vi "3_datatypes.vi"() -> ()   [LabVIEW 2024]
uses:
  class/CalibReport/CalibReport.lvclass
  <vilib>/Python/Open Venv Python Session.vi
panel:
  in  "Datatypes":T1(tab)
  in  "input string":string
  out "result":string
  out "Boolean Output":bool
  in  "Input":bool
  out "Error from python":errorcluster
  in  "List Input":i32[](array[numeric])=[1, 2, 3, 4, 5]
  out "return list":i32[](array[numeric])
  in  "Map":map{string, i32}(c390)
  out "<JSON>":string
  out "CalibPoints":cluster{dbl[], dbl[]}(graph)
  out "__str__ from python object":string
  in  "Temperature [°C]":dbl
  in  "Stop":bool
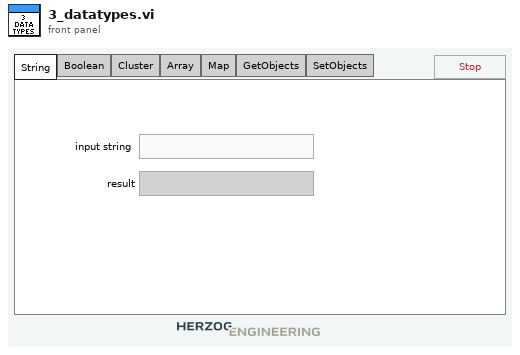
[diagram p1: front panel]
types:
  T1 = enum32{"String", "Boolean", "Cluster", "Array", "Map", "GetObjects", "SetObjects"}
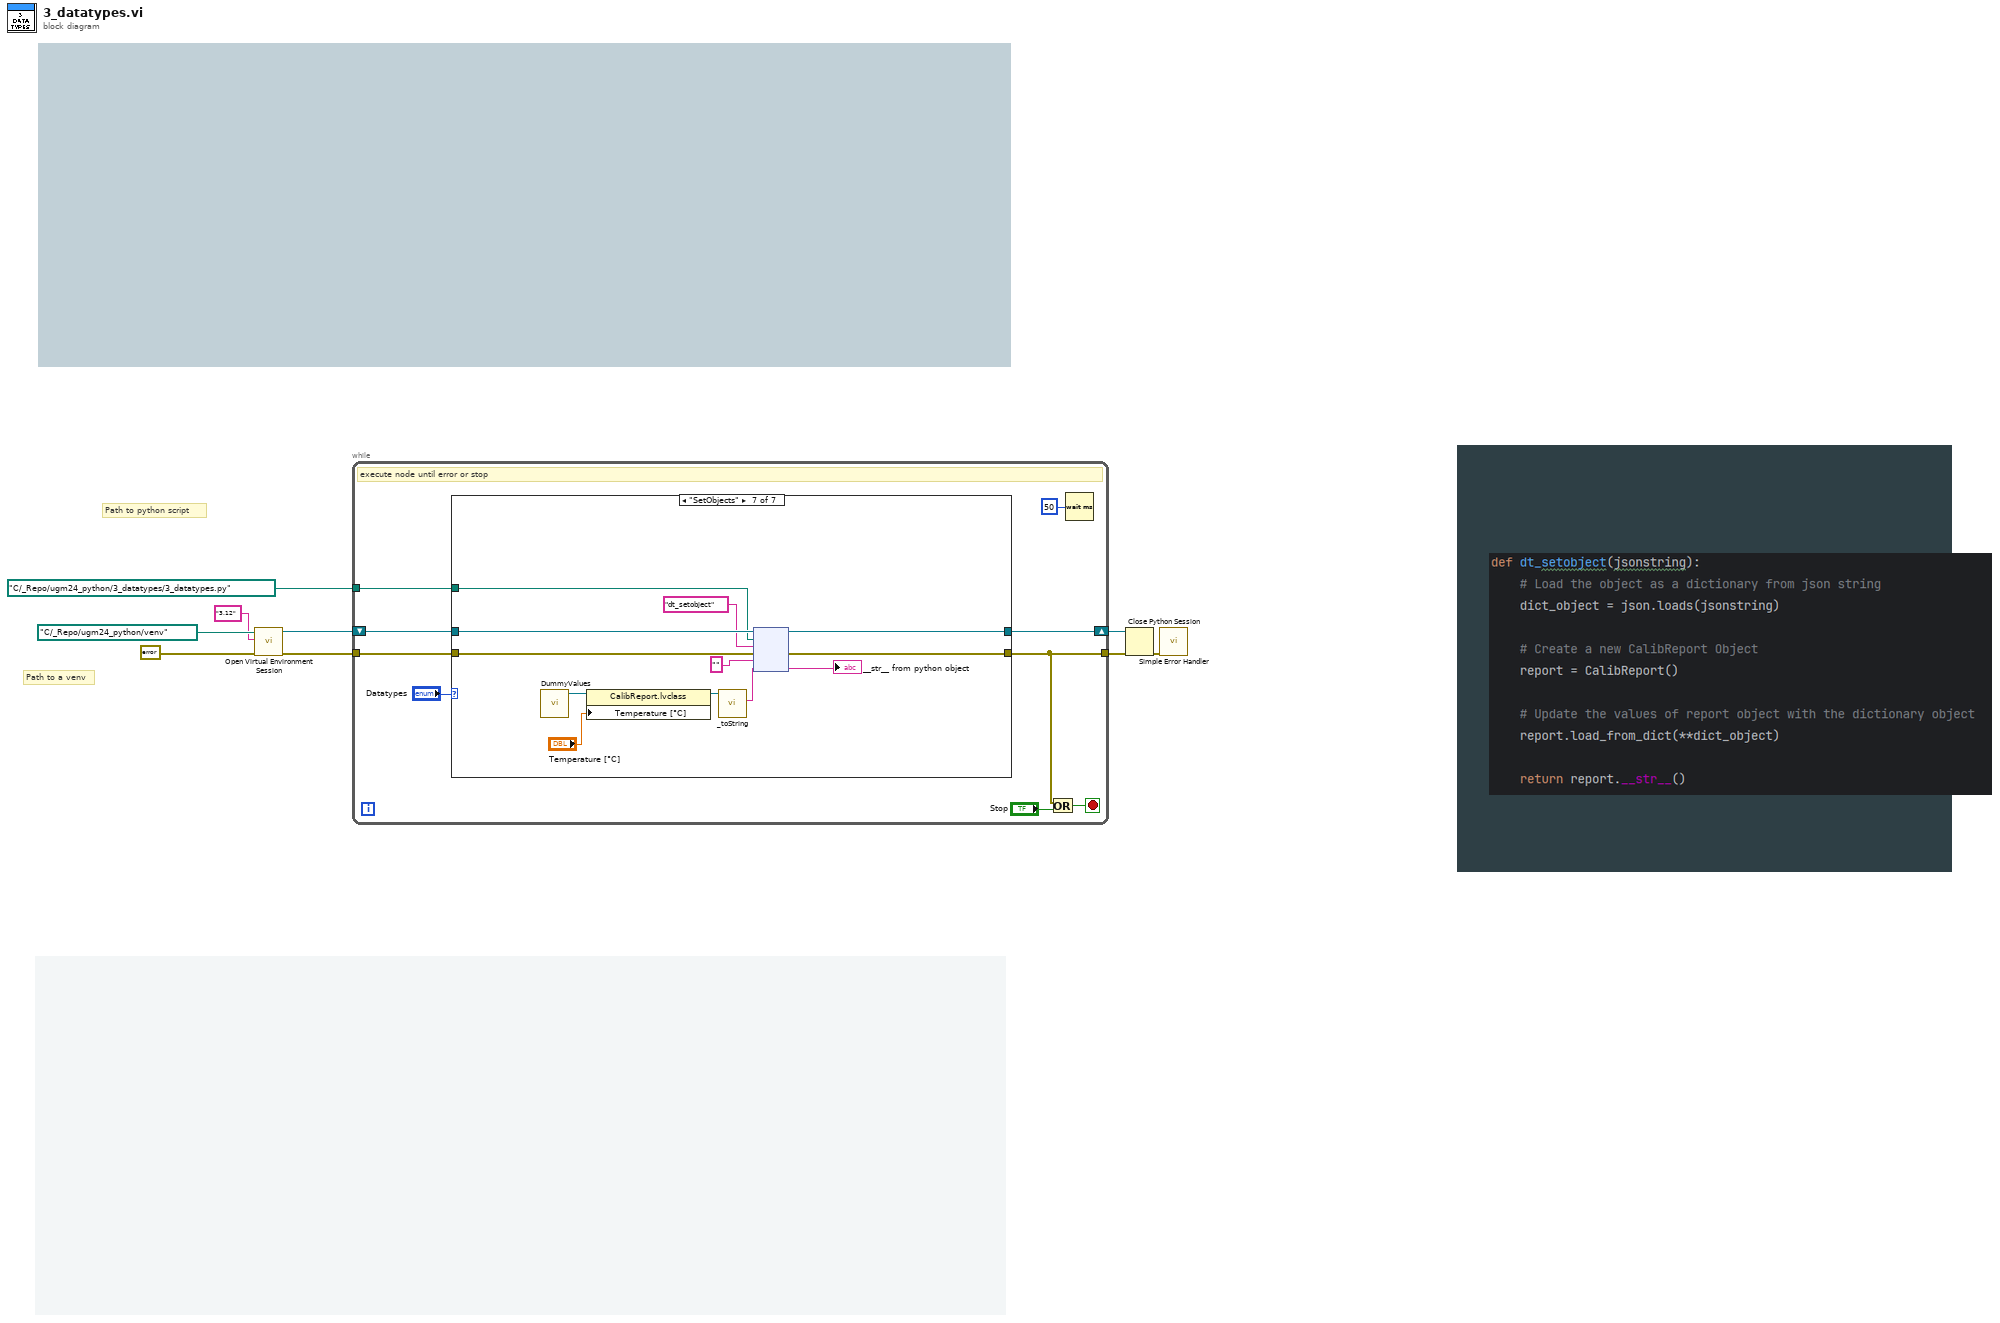
[diagram p0: block diagram]
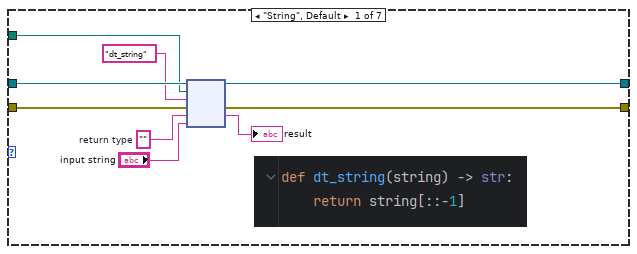
[diagram p2: hidden frame]
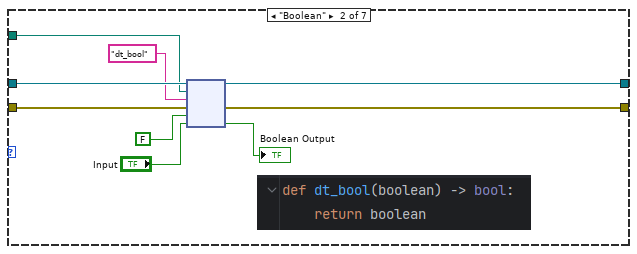
[diagram p3: hidden frame]
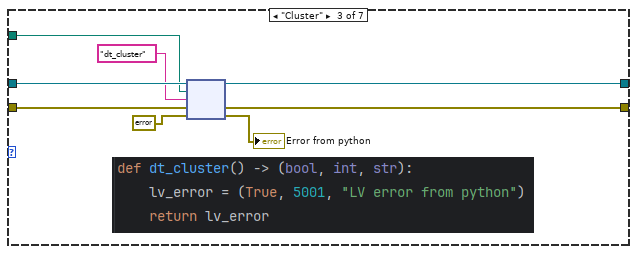
[diagram p4: hidden frame]
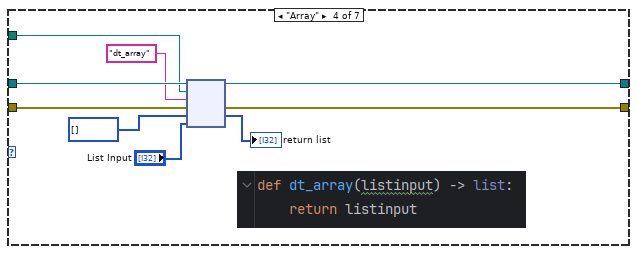
[diagram p5: hidden frame]
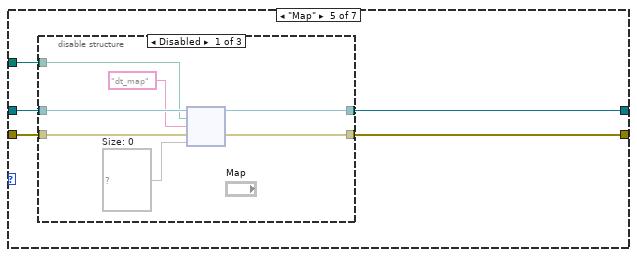
[diagram p6: hidden frame]
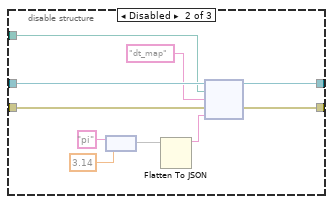
[diagram p7: hidden frame]
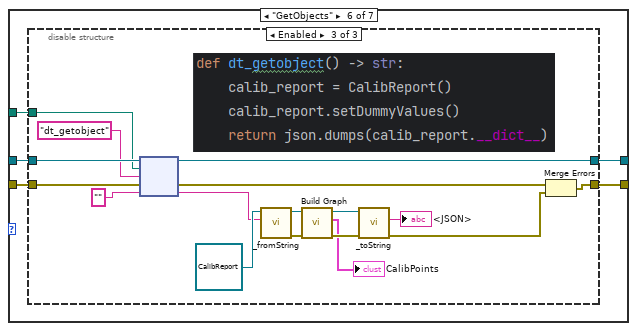
[diagram p9: hidden frame]
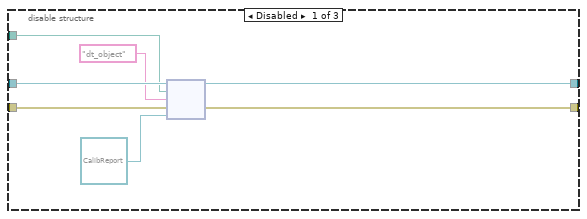
[diagram p10: hidden frame]
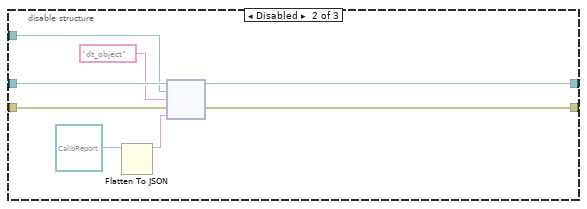
[diagram p11: hidden frame]
diagram:
  # "Path to a venv"
  # "Path to python script"
  n1 = call-poly <vilib>:"Open Virtual Environment Session.vi"("error in (no error)"=errorcluster {"status"=FALSE, "code"=0, "source"=""}, "Python version"="3.12", "Env path"=path "C:/_Repo/ugm24_python/venv") -> ("error out"=w4:errorcluster, "session out"=w3:refnum<k35>)  [unwired: 7 in]
  n2 = while {
    tunnel: w4 -> [w18]
    tunnel: path "C:/_Repo/ugm24_python/3_datatypes/3_datatypes.py" ("Path") -> [w16]
    tunnel: [w13] -> w8
    shift-right: [w12] -> w7
    shift-left: w3 -> [w17]
    stop <- w15 stop-if-true
    # "execute node until error or stop"
    n3 = case shown="\"SetObjects\"" "Datatypes" {
      tunnel: w18 -> [w27 w36 w44 w53 w58 w82 w126]
      tunnel: w17 -> [w26 w35 w43 w52 w57 w81 w125]
      tunnel: w16 -> [w25 w34 w42 w51 w56 w80 w124]
      tunnel: [w21 w32 w40 w49 w55 w79 w123] -> w13
      tunnel: [w20 w31 w39 w48 w54 w78 w122] -> w12
      frame "String", Default {
        w19 = ""  # return type
        n4 = node(w26, w25, "dt_string" ("function name"), w27, w19, "input string") -> (w20:refnum<k35>, w21:errorcluster, →"result":string)  [unwired: 1 in, 2 out]
      }
      frame "Boolean" {
        n5 = node(w35, w34, "dt_bool" ("function name"), w36, FALSE, "Input") -> (w31:refnum<k35>, w32:errorcluster, →"Boolean Output":bool)  [unwired: 1 in, 2 out]
      }
      frame "Cluster" {
        n6 = node(w43, w42, "dt_cluster" ("function name"), w44, errorcluster {"status"=FALSE, "code"=0, "source"=""} ("error in (no error)")) -> (w39:refnum<k35>, w40:errorcluster, →"Error from python":errorcluster)  [unwired: 2 out]
      }
      frame "Array" {
        n7 = node(w52, w51, "dt_array" ("function name"), w53, i32[] [], "List Input") -> (w48:refnum<k35>, w49:errorcluster, →"return list":i32[])  [unwired: 1 in, 2 out]
      }
      frame "Map" {
        n8 = disable-structure shown="Disabled" {
          disable-tunnel: w58 -> [w65 w75 w76]
          disable-tunnel: w57 -> [w64 w74 w77]
          disable-tunnel: w56 -> [w63 w73 _]
          disable-tunnel: [w61 w71 w76] -> w55
          disable-tunnel: [w60 w70 w77] -> w54
          frame Disabled {
            w59 = map{string, i32} {}  # Size: 0
            n9 = node(w64, w63, "dt_map" ("function name"), w65, w59) -> (w60:refnum<k35>, w61:errorcluster)  [unwired: 1 in, 2 out]
          }
          frame Disabled {
            n10 = node("pi" ("key"), 3.14 ("value")) -> (w69:map{string, dbl})
            n11 = Flatten To JSON(anything=w69) -> (JSON string=w66:string)  [unwired: 2 in, 1 out]
            n12 = node(w74, w73, "dt_map" ("function name"), w75, w66) -> (w70:refnum<k35>, w71:errorcluster)  [unwired: 1 in, 2 out]
          }
          frame Enabled {
          }
        }
      }
      frame "GetObjects" {
        n13 = disable-structure shown="Enabled" {
          disable-tunnel: w82 -> [w89 w97 w114]
          disable-tunnel: w81 -> [w88 w96 w113]
          disable-tunnel: w80 -> [w87 w95 w112]
          disable-tunnel: [w85 w93 w99] -> w79
          disable-tunnel: [w84 w92 w109] -> w78
          frame Disabled {
            n14 = node(w88, w87, "dt_object" ("function name"), w89, refnum<class "CalibReport.lvclass"> refnum ("CalibReport.lvclass")) -> (w84:refnum<k35>, w85:errorcluster)  [unwired: 1 in, 2 out]
          }
          frame Disabled {
            n15 = Flatten To JSON(anything=refnum<class "CalibReport.lvclass"> refnum ("CalibReport.lvclass")) -> (JSON string=w90:string)  [unwired: 2 in, 1 out]
            n16 = node(w96, w95, "dt_object" ("function name"), w97, w90) -> (w92:refnum<k35>, w93:errorcluster)  [unwired: 1 in, 2 out]
          }
          frame Enabled {
            n17 = node(w113, w112, "dt_getobject" ("function name"), w114, "") -> (w109:refnum<k35>, w110:errorcluster, w104:string)  [unwired: 2 out]
            n18 = call-dynamic "_fromString.vi"("<JSON>"=w104, "CalibReport in"=refnum<class "CalibReport.lvclass"> refnum) -> ("error out"=w108:errorcluster, "CalibReport out"=w102:refnum<class "CalibReport.lvclass">)  [unwired: 8 in]
            n19 = call-dynamic "Build Graph.vi"("error in (no error)"=w108, "CalibReport in"=w102) -> ("error out"=w103:errorcluster, "CalibPoints"=→"CalibPoints":cluster{dbl[], dbl[]}, "CalibReport out"=w101:refnum<class "CalibReport.lvclass">)  [unwired: 7 in]
            n20 = call-dynamic "_toString.vi"("error in (no error)"=w103, "CalibReport in"=w101) -> ("error out"=w98:errorcluster, "<JSON>"=→"<JSON>":string)  [unwired: 7 in, 1 out]
            n21 = Merge Errors(w110, w98) -> (w99:errorcluster)
          }
        }
      }
      frame "SetObjects" {
        n22 = call "DummyValues.vi"() -> ("CalibReport out"=w119:refnum<class "CalibReport.lvclass">)  [unwired: 10 in, 1 out]
        n23 = property class="CalibReport.lvclass"(reference=w119, "Temperature [°C]"="Temperature [°C]") -> (reference out=w116:refnum<class "CalibReport.lvclass">)  [unwired: 1 in, 1 out]
        n24 = call-dynamic "_toString.vi"("CalibReport in"=w116) -> ("<JSON>"=w118:string)  [unwired: 8 in, 2 out]
        n25 = node(w125, w124, "dt_setobject" ("function name"), w126, "", w118) -> (w122:refnum<k35>, w123:errorcluster, →"__str__ from python object":string)  [unwired: 1 in, 2 out]
      }
    }
    n26 = Or(x=w13, y="Stop") -> (x .or. y?=w15:bool)
    n27 = Wait (ms)(milliseconds to wait=u32 50) -> ()  [unwired: 1 out]
  }
  n28 = Close Python Session(session in=w7, error in=w8) -> (11:w6:errorcluster)
  n29 = call <vilib>:"Simple Error Handler.vi"("error in (no error)"=w6) -> ()  [unwired: 4 in, 5 out]
